vi "Read Configuration File.vi"(8 "error in (no error)":errorcluster, 11 "Instrument in":refnum<class "Instrument.lvclass">) -> (0 "error out":errorcluster, 3 "Instrument out":refnum<class "Instrument.lvclass">)   [LabVIEW 2019, in "Instrument.lvclass"]
uses:
  Instrument.lvclass
  C:/Program Files (x86)/National Instruments/LabVIEW 2019/vi.lib/JKI/JKI SMO/SMO/SMO.lvclass
  Instrument.lvclass/Instrument.ctl
  <userlib>/LevyLab/Configuration/Configuration.lvclass/Configuration.ctl
  <userlib>/LevyLab/Configuration/Write Section.vi
  <vilib>/JKI/JKI SMO/SMO/Protected/ThisLevelClassName.vi
  <userlib>/LevyLab/Configuration/Configuration.lvclass
  4a02a9b6-ced2-4b6e-a21d-b49a582f1553.vi
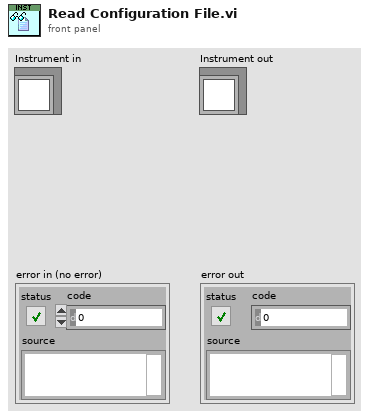
[diagram p1: front panel]
types:
  T1 = typedef "Instrument.lvclass/Configuration--Cluster.ctl" = cluster{"Hardware":T2, "SMO":T3, "Client Type":T5}
  T2 = typedef "Instrument.lvclass/HW Configuration--Cluster.ctl" = cluster{"Address":string, "Type":string, "COM Type":string}
  T3 = typedef "Instrument.lvclass/SMO Configuration--Cluster.ctl" = cluster{"Address":string, "Port":u16, "RC Type":T4, "Debug Mode?":bool, "PGSQL Address":string[], "GetAll Names":string[]}
  T4 = typedef "RemoteControl.lvclass/RC Com Type--enum.ctl" = enum16{"RC", "STM", "ZMQ"}
  T5 = typedef "Instrument.lvclass/Client Type--Enum.ctl" = enum16{"Remote", "Local"}
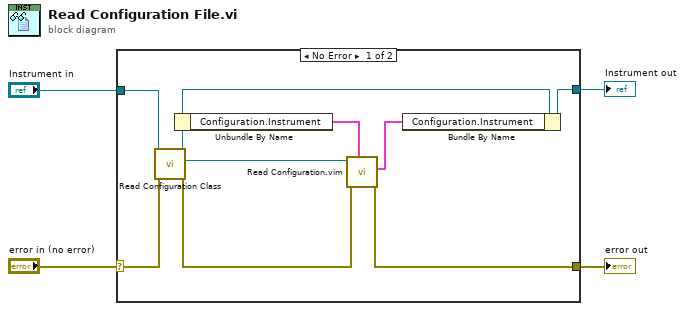
[diagram p0: block diagram]
diagram:
  n1 = case shown="No Error" "error in (no error)" {
    selector: "error in (no error)" -> [w10 w15]
    tunnel: [w5 w15] -> w4
    tunnel: [w13 w14] -> w3
    tunnel: "Instrument in" -> [w12 w14]
    frame No Error {
      n2 = call "Read Configuration Class.vi"("error in (no error)"=w10, "Instrument in"=w12) -> ("error out"=w8:errorcluster, "Configuration"=w7:refnum<class "Configuration.lvclass">, "Instrument out"=w11:refnum<class "Instrument.lvclass">)  [unwired: 7 in]
      n3 = Unbundle By Name(w11) -> ("Configuration.Instrument"=w9:T1)
      n4 = call "Read Configuration.vim"("INI Fomatted Cluster Type"=w9, "error in (no error)"=w8, "Configuration in"=w7) -> ("error out"=w5:errorcluster, "Configuration"=w6:T1)  [unwired: 6 in, 1 out]
      n5 = Bundle By Name(cluster=w11, "Configuration.Instrument"=w6) -> (w13:refnum<class "Instrument.lvclass">)
    }
    frame Error {
    }
  }
  "Instrument out" <- w3
  "error out" <- w4
